vi "AO config not UI to UI.vi"(11 "AO Config":T1 {"output terminal configuration" items=["Default"=-1, "RSE"=10083, "Differential"=10106, "Pseudodifferential"=12529]}) -> (2 "output terminal configuration":i32[](array[numeric]), 3 "AO Config (UI)":T5)   [LabVIEW 2016, in "LockinDAQ.lvclass"]
uses:
  LockinDAQ.lvclass
  Typedefs/AO.config(UI)-array.ctl
  Typedefs/AO.config(UI)-cluster.ctl
  Typedefs/446xAO-enum.ctl
  Typedefs/AO.config-array.ctl
  Typedefs/AO.config-cluster.ctl
  Typedefs/DAQType-enum.ctl
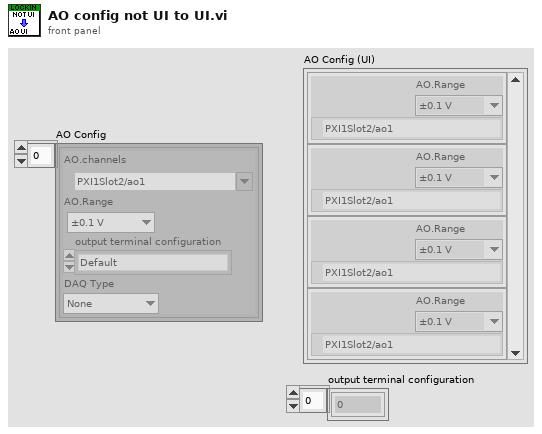
[diagram p1: front panel]
types:
  T1 = typedef "LockinDAQ.lvclass/AO.config-array.ctl" = T2[]
  T2 = typedef "LockinDAQ.lvclass/AO.config-cluster.ctl" = cluster{"AO.channels":tag, "AO.Range":T3, "output terminal configuration":i32, "DAQ Type":T4}
  T3 = typedef "LockinDAQ.lvclass/446xAO-enum.ctl" = enum16{"±0.1 V", "±1.0 V", "±10.0 V"}
  T4 = typedef "LockinDAQ.lvclass/DAQType-enum.ctl" = enum16{"None", "USB 4431", "PXI 446x"}
  T5 = typedef "LockinDAQ.lvclass/AO.config(UI)-array.ctl" = T6[]
  T6 = typedef "LockinDAQ.lvclass/AO.config(UI)-cluster.ctl" = cluster{"AO.Range":T3, "AO.channels":tag}
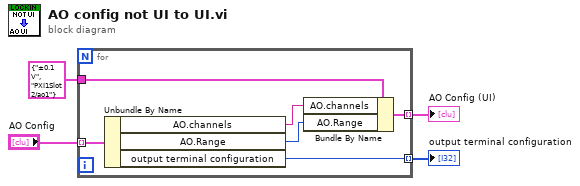
[diagram p0: block diagram]
diagram:
  n1 = for {
    tunnel: T6 {"AO.Range"=enum."±0.1 V", "AO.channels"="PXI1Slot2/ao1"} ("Cluster") -> [w10]
    tunnel: "AO Config" -> [w9] mode=indexing
    tunnel: [w6] -> w2 mode=indexing
    tunnel: [w5] -> w1 mode=indexing
    n2 = Unbundle By Name(w9) -> ("AO.channels"=w8:tag, "AO.Range"=w7:T3, "output terminal configuration"=w5:i32)
    n3 = Bundle By Name(cluster=w10, "AO.channels"=w8, "AO.Range"=w7) -> (w6:T6)
  }
  "AO Config (UI)" <- w2
  "output terminal configuration" <- w1
